vi "Read.vi"(8 "error in":errorcluster, 11 "VISA resource name in":refnum<visa-resource-name>) -> (0 "error out":errorcluster, 2 "Value":dbl, 3 "VISA resource name out":refnum<visa-resource-name>)   [LabVIEW 2021, in "Keysight U1282A.lvlib"]
doc: "El comando de lectura (READ?) regresa un valor despues de un cyclo de redisparo (re-trigger) cuando el instrumento está en Trigger Hold mode. Cuando el instrumento no esta en Trigger Hold mode, este comando regresa el valor en la pantalla del instrumento."
uses:
  Keysight U1282A.lvlib
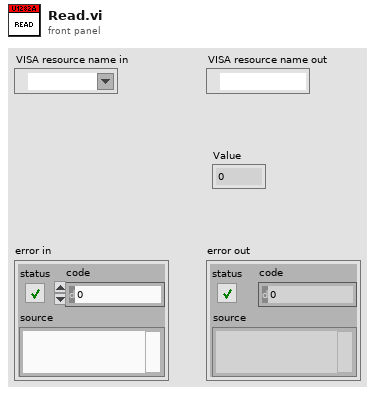
[diagram p1: front panel]
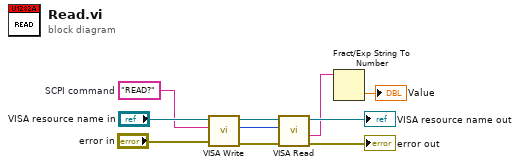
[diagram p0: block diagram]
diagram:
  w5 = "READ?"  # SCPI command
  n1 = call "VISA Write.vi"("error in"="error in", "SCPI command"=w5, "VISA resource in"="VISA resource name in") -> ("error out"=w9:errorcluster, "Bytes at Port out"=w3:u32, "VISA resource out"=w4:refnum<visa-resource-name>)  [unwired: 6 in]
  n2 = call "VISA Read.vi"("error in"=w9, "Bytes at Port in"=w3, "VISA resource in"=w4) -> ("error out"=→"error out":errorcluster, "Reading"=w2:string, "VISA resource out"=→"VISA resource name out":refnum<visa-resource-name>)  [unwired: 5 in, 1 out]
  n3 = Fract/Exp String To Number(string=w2) -> (number=→"Value":dbl)  [unwired: 3 in, 1 out]
